vi "HW3_2017_BEEP.vi"() -> ()   [LabVIEW 2017]
panel:
  in  "min":dbl
  in  "hour":dbl
  in  "OK Button":bool
  out "Boolean":bool
  in  "SET ALARM":bool
  out "ALARMING TIME":string
  out "DATE":string
  in  "reinstate":bool
  in  "sec":dbl
  in  "min":dbl
  in  "hour":dbl
  in  "reset":bool
  out "sec":dbl(knob) scale=0.0..60.0
  out "min":dbl(knob) scale=0.0..60.0
  out "hour":dbl(knob) scale=0.0..12.0
  in  "stop":bool
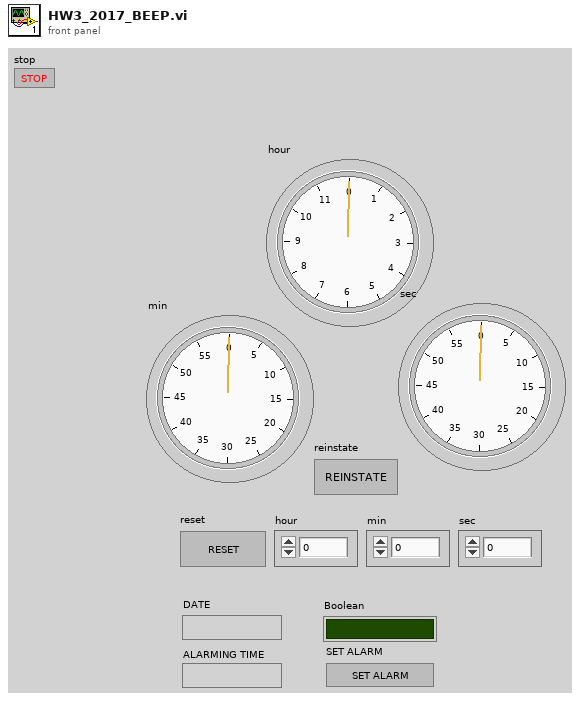
[diagram p1: front panel]
types:
  T1 = typedef "LVDateTimeRec.ctl" = cluster{"fractional second":dbl, "second":i32, "minute":i32, "hour":i32, "day of month":i32, "month":i32, "year":i32, "day of week":i32, "day of year":i32, "DST":i32}
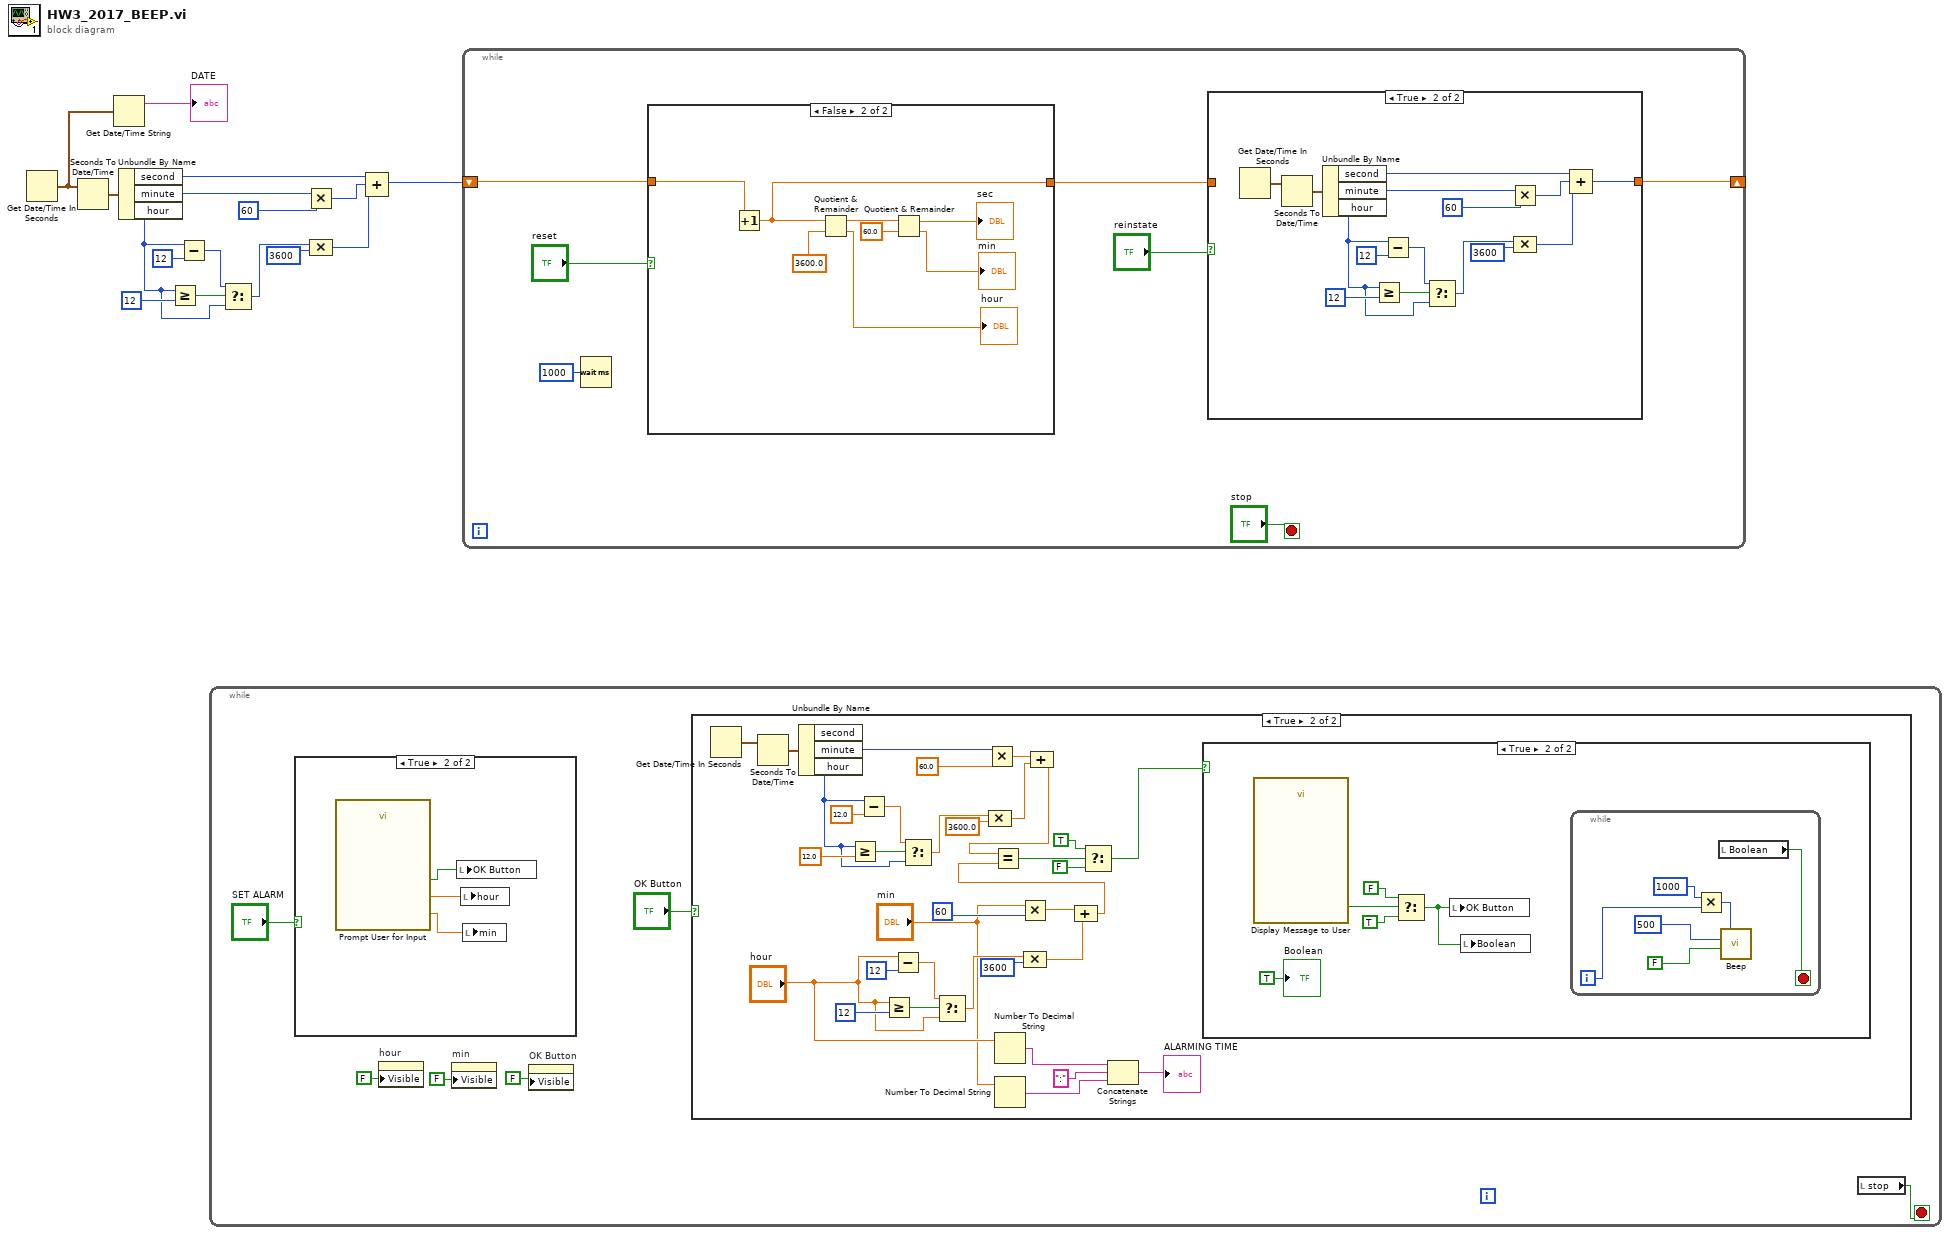
[diagram p0: block diagram]
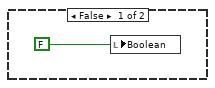
[diagram p3: hidden frame]
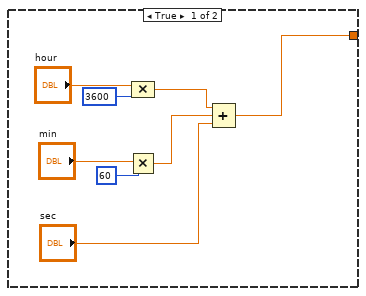
[diagram p6: hidden frame]
diagram:
  n1 = Get Date/Time In Seconds() -> (seconds since 1Jan1904=w5:timestamp)
  n2 = Seconds To Date/Time(time stamp (now)=w5) -> (date time rec=w14:T1)  [unwired: 1 in]
  n3 = Get Date/Time String(seconds (now)=w5) -> (date string=→"DATE":string)  [unwired: 2 in, 1 out]
  n4 = Unbundle By Name(w14) -> ("second"=w12:i32, "minute"=w13:i32, "hour"=w7:i32)
  n5 = Greater Or Equal?(x=w7, y=12) -> (x >= y?=w10:bool)
  n6 = Subtract(x=w7, y=12) -> (x-y=w8:i32)
  n7 = while {
    stop <- w18 stop-if-true
    n8 = case shown="True" "SET ALARM" {
      frame False {
      }
      frame True {
        n9 = call "Prompt User for Input"() -> ("Minute"=w71:dbl, "Hour"=w70:dbl, "OK"=w69:bool)  [unwired: 16 in, 1 out]
        n10 = local write "OK Button"(w69) -> ()
        n11 = local write "hour"(w70) -> ()
        n12 = local write "min"(w71) -> ()
      }
    }
    n13 = property on="hour" class="DigNum (strict)"("Visible"=FALSE) -> ()  [unwired: 2 in, 2 out]
    n14 = property on="min" class="DigNum (strict)"("Visible"=FALSE) -> ()  [unwired: 2 in, 2 out]
    n15 = property on="OK Button" class="Bool (strict)"("Visible"=FALSE) -> ()  [unwired: 2 in, 2 out]
    n16 = case shown="True" "OK Button" {
      frame False {
      }
      frame True {
        n17 = Get Date/Time In Seconds() -> (seconds since 1Jan1904=w26:timestamp)
        n18 = Seconds To Date/Time(time stamp (now)=w26) -> (date time rec=w29:T1)  [unwired: 1 in]
        n19 = Unbundle By Name(w29) -> ("minute"=w30:i32, "hour"=w23:i32)  [unwired: 1 out]
        n20 = Greater Or Equal?(x=w23, y=12.0) -> (x >= y?=w32:bool)
        n21 = Subtract(x=w23, y=12.0) -> (x-y=w34:dbl)
        n22 = Greater Or Equal?(x="hour", y=12) -> (x >= y?=w51:bool)
        n23 = Subtract(x="hour", y=12) -> (x-y=w49:dbl)
        n24 = Select(t=w34, s=w32, f=w23) -> (s? t:f=w35:dbl)
        n25 = Select(t=w49, s=w51, f="hour") -> (s? t:f=w48:dbl)
        n26 = Multiply(x=w30, y=60.0) -> (x*y=w36:dbl)
        n27 = Compound Arithmetic op=MULTIPLY(w35, 3600.0) -> (w37:dbl)
        n28 = Number To Decimal String(number="hour") -> (decimal integer string=w43:string)  [unwired: 1 in]
        n29 = Number To Decimal String(number="min") -> (decimal integer string=w41:string)  [unwired: 1 in]
        n30 = Multiply(x="min", y=60) -> (x*y=w54:dbl)
        n31 = Compound Arithmetic op=MULTIPLY(w48, 3600) -> (w53:dbl)
        n32 = Compound Arithmetic op=ADD(w36, w37) -> (w25:dbl)
        n33 = Compound Arithmetic op=ADD(w54, w53) -> (w47:dbl)
        n34 = Equal?(x=w25, y=w47) -> (x = y?=w46:bool)
        n35 = Select(t=TRUE, s=w46, f=FALSE) -> (s? t:f=w24:bool)
        n36 = Concatenate Strings(w43, ":", w41) -> (→"ALARMING TIME":string)
        n37 = case shown="True" w24 {
          frame False {
            n38 = local write "Boolean"(FALSE ("Boolean")) -> ()
          }
          frame True {
            n39 = call "Display Message to User"() -> ("OK"=w58:bool)  [unwired: 10 in, 1 out]
            n40 = Select(t=FALSE ("Boolean"), s=w58, f=TRUE) -> (s? t:f=w59:bool)
            n41 = local write "OK Button"(w59) -> ()
            n42 = local write "Boolean"(w59) -> ()
            n43 = while {
              i -> [w64]
              stop <- w63 stop-if-true
              n44 = Multiply(x=u32 1000 ("frequency (Hz)"), y=w64) -> (x*y=w68:u32)
              n45 = local read "Boolean"() -> (w63:bool)
              n46 = call <vilib>:"Beep.vi"("use system alert? (T)"=FALSE, "duration (msec)"=u32 500, "frequency (Hz)"=w68) -> ()  [unwired: 9 in]
            }
            "Boolean" <- TRUE ("Boolean")
          }
        }
      }
    }
    n47 = local read "stop"() -> (w18:bool)
  }
  n48 = Select(t=w8, s=w10, f=w7) -> (s? t:f=w6:i32)
  n49 = Multiply(x=w13, y=60) -> (x*y=w2:i32)
  n50 = Compound Arithmetic op=MULTIPLY(w6, 3600) -> (w1:i32)
  n51 = Compound Arithmetic op=ADD(w12, w2, w1) -> (w4:i32)
  n52 = while {
    shift-right: [w73] -> _
    shift-left: w4 -> [w77]
    stop <- "stop" stop-if-true
    n53 = Wait (ms)(milliseconds to wait=u32 1000) -> ()  [unwired: 1 out]
    n54 = case shown="False" "reset" {
      tunnel: w77 -> [_ w110]
      tunnel: [w95 w103] -> w74
      frame True {
        n55 = Multiply(x="min", y=60) -> (x*y=w97:dbl)
        n56 = Compound Arithmetic op=MULTIPLY("hour", 3600) -> (w98:dbl)
        n57 = Compound Arithmetic op=ADD(w98, w97, "sec") -> (w95:dbl)
      }
      frame False {
        n58 = Increment(x=w110) -> (x+1=w103:dbl)
        n59 = Quotient & Remainder(x=w103, y=3600.0) -> (x-y*floor(x/y)=w108:dbl, floor(x/y)=→"hour":dbl)
        n60 = Quotient & Remainder(x=w108, y=60.0) -> (x-y*floor(x/y)=→"sec":dbl, floor(x/y)=→"min":dbl)
      }
    }
    n61 = case shown="True" "reinstate" {
      tunnel: w74 -> [w79 _]
      tunnel: [w79 w80] -> w73
      frame False {
      }
      frame True {
        n62 = Get Date/Time In Seconds() -> (seconds since 1Jan1904=w91:timestamp)
        n63 = Seconds To Date/Time(time stamp (now)=w91) -> (date time rec=w90:T1)  [unwired: 1 in]
        n64 = Unbundle By Name(w90) -> ("second"=w87:i32, "minute"=w89:i32, "hour"=w82:i32)
        n65 = Greater Or Equal?(x=w82, y=12) -> (x >= y?=w85:bool)
        n66 = Subtract(x=w82, y=12) -> (x-y=w83:i32)
        n67 = Select(t=w83, s=w85, f=w82) -> (s? t:f=w81:i32)
        n68 = Multiply(x=w89, y=60) -> (x*y=w92:i32)
        n69 = Compound Arithmetic op=MULTIPLY(w81, 3600) -> (w88:i32)
        n70 = Compound Arithmetic op=ADD(w87, w92, w88) -> (w80:i32)
      }
    }
  }
